vi "Start Server.vi"(5 "Server Key File (.key)":path, 7 "Server Certificate File (.crt)":path, 8 "error in (no error)":errorcluster, 10 "Server Id":T1, 11 "Server Address":string) -> (0 "error out":errorcluster, 2 "Listening Port":i32, 3 "Server Id Out":T1)   [LabVIEW 2019, in "Template Client.lvlib" / "gprc-lvsupport.lvlib"]
uses:
  gprc-lvsupport.lvlib
  typeDefs/grpcId.ctl
  <vilib>/Utility/error.llb/Error Cluster From Error Code.vi
  <vilib>/ErrorRing/Error Ring.xnode
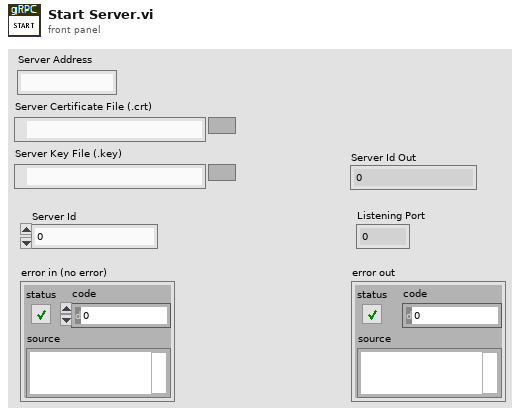
[diagram p1: front panel]
types:
  T1 = typedef "Template Client.lvlib/gprc-lvsupport.lvlib/grpcId.ctl" = u64
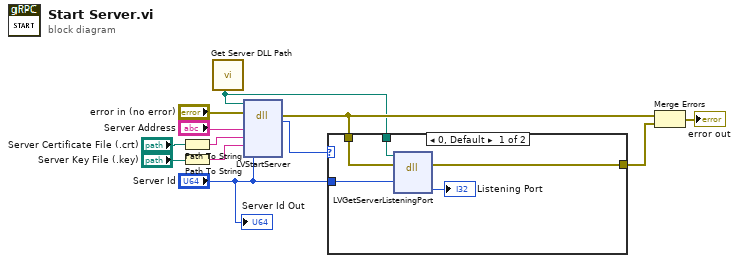
[diagram p0: block diagram]
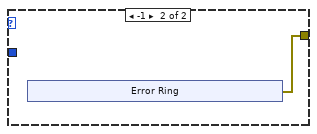
[diagram p2: hidden frame]
diagram:
  n1 = Path To String(path="Server Certificate File (.crt)") -> (string=w10:string)
  n2 = Path To String(path="Server Key File (.key)") -> (string=w9:string)
  n3 = call "Get Server DLL Path.vi"() -> ("Server dll path"=w2:path)
  n4 = dll-call lib="?" fn="LVStartServer"(path in=w2, error in="error in (no error)", "serveraddress"="Server Address", "serverCertificateFile"=w10, "serverKeyFile"=w9, "serverid"="Server Id") -> (error out=w3:errorcluster, "return type"=w6:i32)  [unwired: 5 in, 1 out]
  n5 = case shown="0, Default" w6 {
    tunnel: [w17 w18] -> w4
    tunnel: w3 -> [w16 _]
    tunnel: w2 -> [w15 _]
    tunnel: "Server Id" -> [w14 _]
    frame 0, Default {
      n6 = dll-call lib="?" fn="LVGetServerListeningPort"(path in=w15, error in=w16, "serverId"=w14) -> (error out=w17:errorcluster, "listeningPort"=→"Listening Port":i32)  [unwired: 4 in, 1 out]
    }
    frame -1 {
      n7 = xnode "Error Ring"() -> ("error out"=w18:errorcluster)
    }
  }
  n8 = Merge Errors(w3, w4) -> (→"error out":errorcluster)
  "Server Id Out" <- "Server Id"
